vi "Send OOB RX.vi"(8 "error in (no error)":errorcluster, 11 "CIFTemplatePlugin in":refnum<class "TemplatePlugin.lvclass">) -> (0 "error out":errorcluster, 3 "CIFTemplatePlugin out":refnum<class "TemplatePlugin.lvclass">)   [LabVIEW 2021, in "TemplatePlugin.lvclass"]
uses:
  TemplatePlugin.lvclass
  TemplatePlugin.lvclass/TemplatePlugin.ctl
  CIF-LVCore/src/CIFCore/Class/CIFCorePlugin.lvclass
  OOB/OOB_Rx/TemplateOOB_Rx.lvclass
  D:/dev/CIF-LVCore/src/CIFCore/Class/CIFCorePlugin.lvclass
  D:/dev/Plugins/Template/Class/TemplatePlugin.lvclass
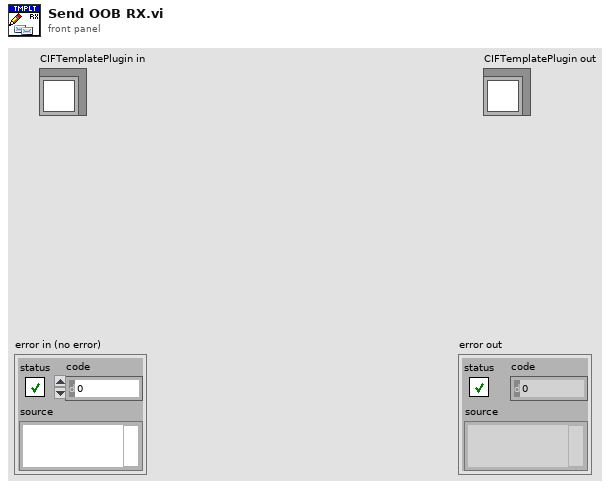
[diagram p1: front panel]
types:
  T1 = typedef "TemplateOOB_Rx.lvclass/Cyclic Data.ctl" = cluster{"Numeric":i32}
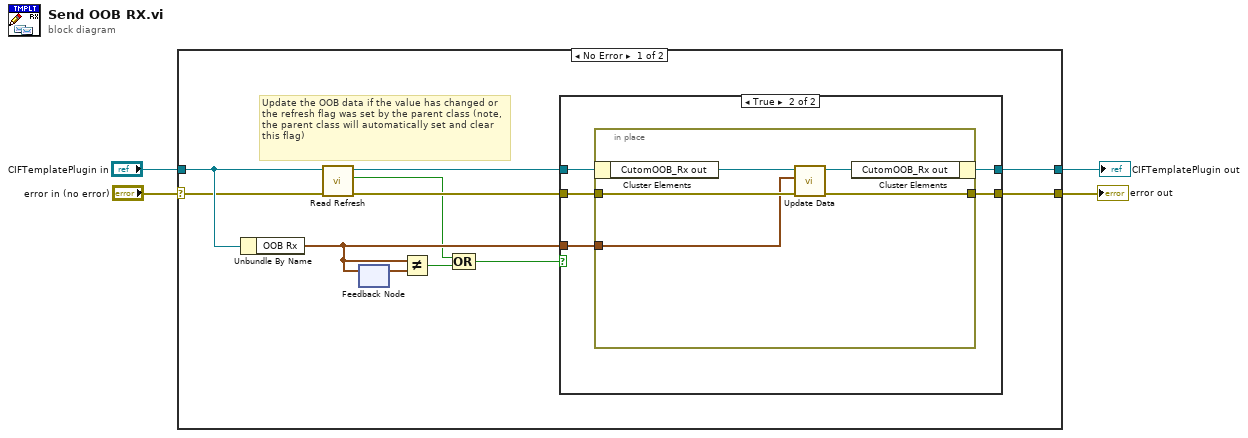
[diagram p0: block diagram]
diagram:
  n1 = case shown="No Error" "error in (no error)" {
    selector: "error in (no error)" -> [w8 w29]
    tunnel: [w10 w29] -> w3
    tunnel: [w11 w28] -> w1
    tunnel: "CIFTemplatePlugin in" -> [w9 w28]
    frame No Error {
      # "Update the OOB data if the value has changed or the refresh flag was set by the parent class (note, the parent class will automatically set and clear this flag)"
      n2 = Unbundle By Name(w9) -> ("OOB Rx"=w13:T1)
      n3 = call "Read Refresh.vi"("error in (no error)"=w8, "CIFCorePlugin in"=w9) -> ("error out"=w6:errorcluster, "Refresh"=w5:bool, "CIFCorePlugin out"=w7:refnum<class "TemplatePlugin.lvclass">)  [unwired: 7 in]
      n4 = feedback-in #1(w13) -> ()
      n5 = feedback #1() -> (w15:T1)  [unwired: 1 in]
      n6 = Not Equal?(x=w13, y=w15) -> (x != y?=w14:bool)
      n7 = Compound Arithmetic op=OR(w5, w14) -> (w12:bool)
      n8 = case shown="True" w12 {
        tunnel: w6 -> [w16 w22]
        tunnel: w7 -> [w17 w21]
        tunnel: w13 -> [_ w20]
        tunnel: [w17 w19] -> w11
        tunnel: [w16 w18] -> w10
        frame False {
        }
        frame True {
          n9 = in-place {
            in-place-border: w22 -> [w26]
            in-place-border: [w24] -> w18
            in-place-border: w20 -> [w23]
            n10 = in-place-cluster #2(w21) -> ("CutomOOB_Rx out"=w27:refnum<class "TemplateOOB_Rx.lvclass">)
            n11 = call "Update Data.vi"("error in"=w26, "Data"=w23, "CutomOOB_Rx in"=w27) -> ("error out"=w24:errorcluster, "CutomOOB_Rx out"=w25:refnum<class "TemplateOOB_Rx.lvclass">)  [unwired: 7 in]
            n12 = in-place-cluster #2("CutomOOB_Rx out"=w25) -> (w19:refnum<class "TemplatePlugin.lvclass">)
          }
        }
      }
    }
    frame Error {
    }
  }
  "error out" <- w3
  "CIFTemplatePlugin out" <- w1
